vi "Archive Graduated Students from Provided List.vi"() -> ()   [LabVIEW 2019]
uses:
  <vilib>/Utility/file.llb/Read Delimited Spreadsheet (string).vi
panel:
  in  "END CODE":bool
  out "Students who still have items and were not archived":string[](array[string])
  in  "Archive Users":bool
  out "BYU ID # List In":string[](array[string])
  in  "Load List":bool
  in  "List of BYU ID #'s":path
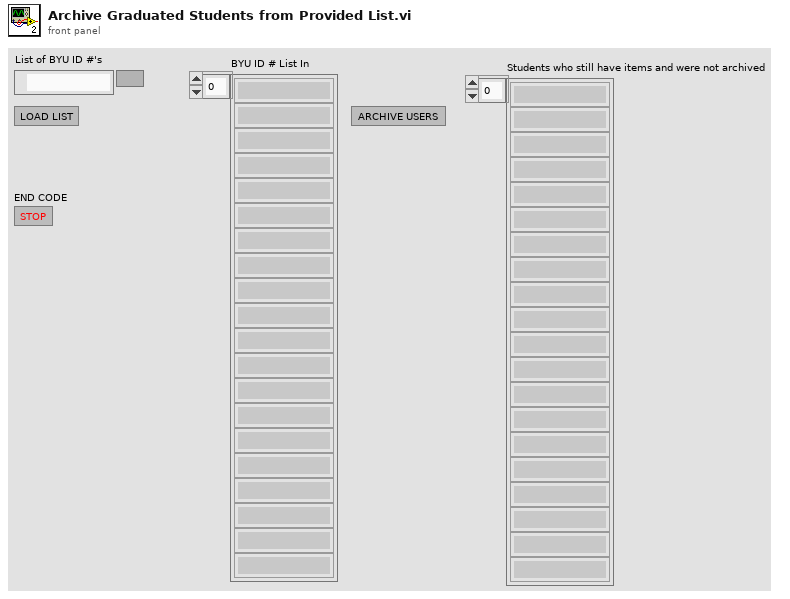
[diagram p1: front panel]
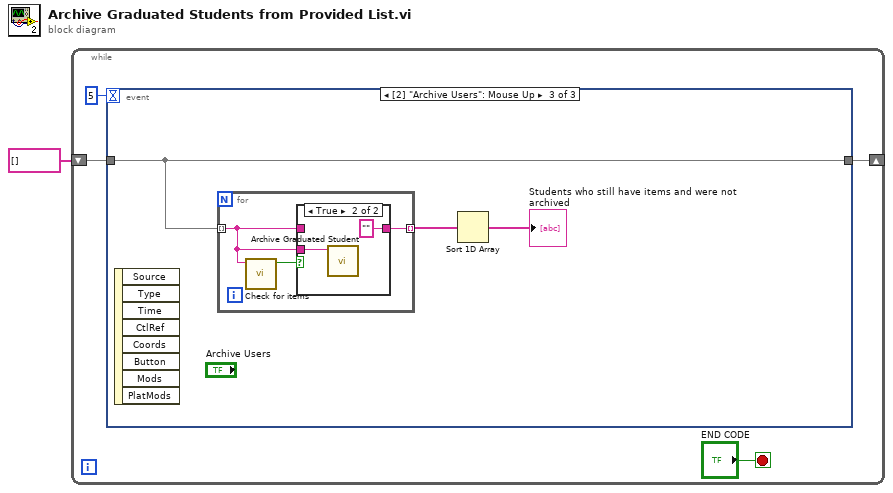
[diagram p0: block diagram]
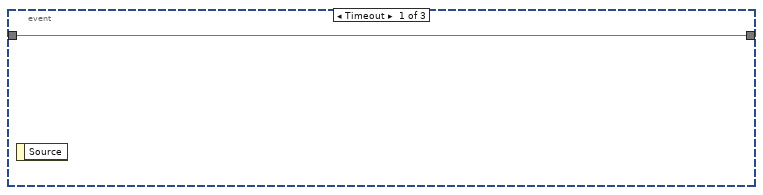
[diagram p2: hidden frame]
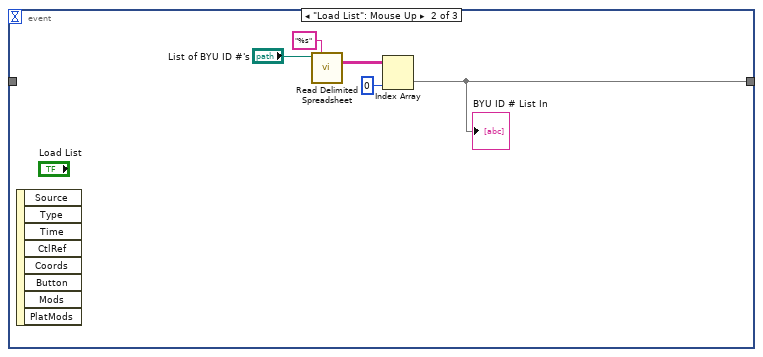
[diagram p3: hidden frame]
diagram:
  n1 = while {
    shift-right: [w3] -> _
    shift-left: string[] [] ("BYU ID # List In") -> [w4]
    stop <- "END CODE" stop-if-true
    n2 = event shown="[2] \"Archive Users\": Mouse Up" {
      selector: _ -> [_ _ _]
      dyn-events: _ -> [_ _ _]
      timeout: 5 -> [_ _ _]
      tunnel: w4 -> [w6 _ w14]
      tunnel: [w6 w7 w14] -> w3
      event Timeout {
        n3 = event-data() -> ()  [unwired: 1 in, 1 out]
      }
      event "Load List": Mouse Up {
        n4 = event-data() -> ()  [unwired: 1 in, 8 out]
        n5 = call-poly <vilib>:"Read Delimited Spreadsheet.vi"("file path (dialog if empty)"="List of BYU ID #'s", "format (%s)"="%s" ("format (%.3f)")) -> ("all rows"=w9:string[][])  [unwired: 8 in, 5 out]
        n6 = Index Array(array=w9, index (col)=0 ("disabled index (col)")) -> (element=w7:string[])  [unwired: 1 in]
        "BYU ID # List In" <- w7
      }
      event "Archive Users": Mouse Up {
        n7 = event-data() -> ()  [unwired: 1 in, 8 out]
        n8 = for {
          tunnel: w14 -> [w15] mode=indexing
          tunnel: [w16] -> w13 mode=indexing
          n9 = call "Check for items.vi"("BYU ID # In"=w15) -> ("No Items"=w17:bool)  [unwired: 10 in]
          n10 = case shown="True" w17 {
            tunnel: w15 -> [w18 _]
            tunnel: [w18 "" ("String")] -> w16
            tunnel: w15 -> [_ w19]
            frame False {
            }
            frame True {
              n11 = call "Archive Graduated Student.vi"("BYU ID # In"=w19) -> ()  [unwired: 11 in]
            }
          }
        }
        n12 = Sort 1D Array(array=w13) -> (sorted array=→"Students who still have items and were not archived":string[])
      }
    }
  }
